vi "Set configuration chain.vi"(8 "error in (no error)":errorcluster, 9 "class names":string[](array[string]), 10 "configuration":variant[](array[variant]), 11 "ConfocalStage in":refnum<class "ConfocalStage.lvclass">) -> (0 "error out":errorcluster, 3 "ConfocalStage out":refnum<class "ConfocalStage.lvclass">)   [LabVIEW 2012, in "ConfocalStage.lvclass"]
uses:
  ConfocalStage.lvclass
  <vilib>/Distrio/Murmex/Murmex/Murmex.lvclass
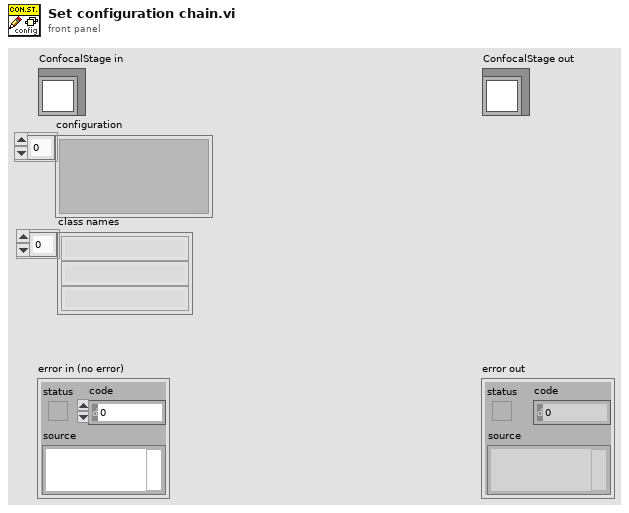
[diagram p1: front panel]
types:
  T1 = typedef "ConfocalStage.lvclass/configuration.ctl" = cluster{"startup speed":dbl[unit], "Serial port":cluster{"baud rate":u32, "data bits":u16, "parity (0:none)":enum16{"None", "Odd", "Even", "Mark", "Space"}, "flow control":u16, "stop bits":u16, "termination char":u8, "send termination char?":bool, "COM port":refnum<visa-resource-name>}, "accelleration ramp":dbl[unit], "speed conversion":dbl, "position conversion X":dbl, "position conversion Y":dbl, "position conversion Z":dbl}
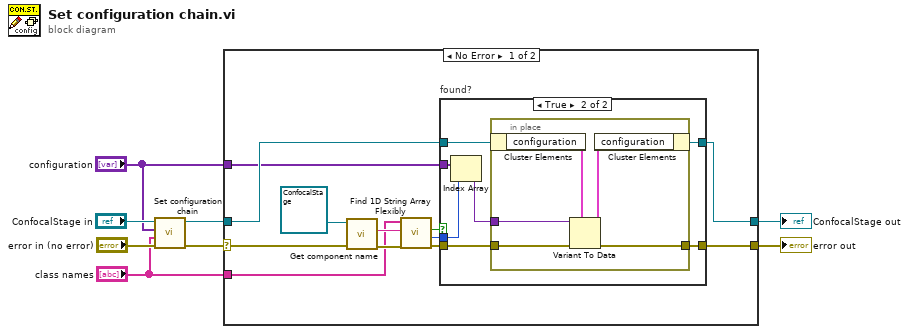
[diagram p0: block diagram]
diagram:
  n1 = call-parent "Set configuration chain.vi"("error in (no error)"="error in (no error)", "class names"="class names", "configuration"="configuration", "Murmex in"="ConfocalStage in") -> ("error out"=w6:errorcluster, "Murmex out"=w3:refnum<class "ConfocalStage.lvclass">)  [unwired: 6 in]
  n2 = case shown="No Error" w6 {
    selector: w6 -> [w15 w36]
    tunnel: [w14 w36] -> w5
    tunnel: [w12 w35] -> w4
    tunnel: w3 -> [w13 w35]
    tunnel: "configuration" -> [w11 _]
    tunnel: "class names" -> [w10 _]
    frame No Error {
      n3 = call <vilib>:"Get component name.vi"("error in (no error)"=w15, "Murmex in"=refnum<class "ConfocalStage.lvclass"> refnum ("ConfocalStage in")) -> ("error out"=w20:errorcluster, "component name"=w19:string)  [unwired: 7 in, 1 out]
      n4 = call <vilib>:"Find 1D String Array Flexibly.vi"("error in (no error)"=w20, "element"=w19, "array"=w10) -> ("error out"=w18:errorcluster, "index of element"=w16:i32, "found?"=w17:bool)  [unwired: 6 in]
      n5 = case "found?" shown="True" w17 {
        tunnel: w11 -> [_ w29]
        tunnel: w13 -> [w22 w27]
        tunnel: [w22 w26] -> w12
        tunnel: [w21 w25] -> w14
        tunnel: w18 -> [w21 w24]
        tunnel: w16 -> [_ w23]
        frame False {
        }
        frame True {
          n6 = Index Array(array=w29, index=w23) -> (element=w28:variant)
          n7 = in-place {
            in-place-border: w28 -> [w34]
            in-place-border: w24 -> [w32]
            in-place-border: [w30] -> w25
            n8 = in-place-cluster #1(w27) -> ("configuration"=w33:T1)
            n9 = Variant To Data(error in=w32, type=w33, Variant=w34) -> (data=w31:T1, error out=w30:errorcluster)
            n10 = in-place-cluster #1("configuration"=w31) -> (w26:refnum<class "ConfocalStage.lvclass">)
          }
        }
      }
    }
    frame Error {
    }
  }
  "error out" <- w5
  "ConfocalStage out" <- w4
